vi "PythonIDE 2.vi"(7 "Python version":string="3.9", 11 "Port":string) -> ()   [LabVIEW 2020]
uses:
  <vilib>/event_ctls.llb/eventvkey.ctl
  <vilib>/Utility/error.llb/DialogType.ctl
  Serial_Global.vi
panel:
  out "VKey":T1
  out "message":string=" INSTRUCTIONS:\r\rNormal Use:  When using subVIs that incorporate the error in/error out (or error I/O) structure, place this handler where you want to inform the user of an error, typically at the end of the I/O data path, as the last action of the program.  If the error in error? is ERROR, the handler creates a message describing the error and its source.  If the type of dialog = 1 (default), the message is displayed to the user, who can only acknowedge it.  If the type = 2, the user can acknowledge the message or abort execution; aborting a program with active I/O is not recommended.  If the type = 0, no message is displayed; this is used to process the error programmatically, and the error out cluster elements are wired to individual terminals for that reason.  \r\rOther Use:\n\r\nlocal testing.  To test the error code of a subVI or function that does not have the error I/O structure, you can wire its error code and a source string to the local error code and error source inputs.  If error in error? indicates no error and error code is not equal to 0, the local code and source are substituted for the error in values, and error? is set TRUE (ERROR)."
  in  "Browser":bool
  in  "Name":string="code.py"
  in  "Save SPIKE":bool
  in  "Save PC":bool
  out "Script":string
  in  "Python Code":string
  out "Console":string
  in  "stop":bool
  in  "Ctrl C":bool
  in  "run":bool
  # "PyVIEW IDE\nversion 0.1b03"
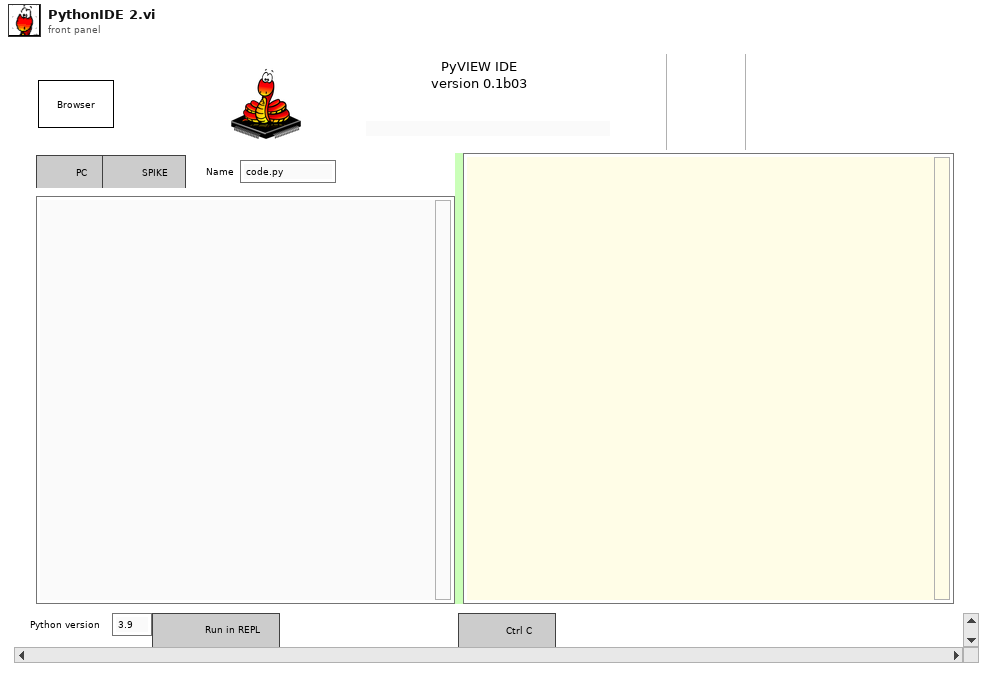
[diagram p1: front panel]
types:
  T1 = typedef "eventvkey.ctl" = enum16{"ASCII", "Enter", "Return", "Shift", "Ctrl", "Alt", "Cmd", "Opt", "Caps", "NumLock", "Clear", "Break", "Up", "Down", "Left", "Right", "Insert", "Delete", "Home", "End", "PageUp", "PageDown", "Escape", "Help", "Pause", "ScrollLock", "F1", "F2", "F3", "F4", "F5", "F6", "F7", "F8", "F9", "F10", "F11", "F12", "F13", "F14", "F15", "F16", "F17", "F18", "F19", "F20", "F21", "F22", "F23", "F24", "Play", "VolumeUp", "VolumeDown", "Mute", "Two Byte Char"}
  T2 = typedef "PythonCtrl.ctl" = cluster{"session":refnum<k35>, "PyPath":path}
  T3 = typedef "DialogType.ctl" = u16
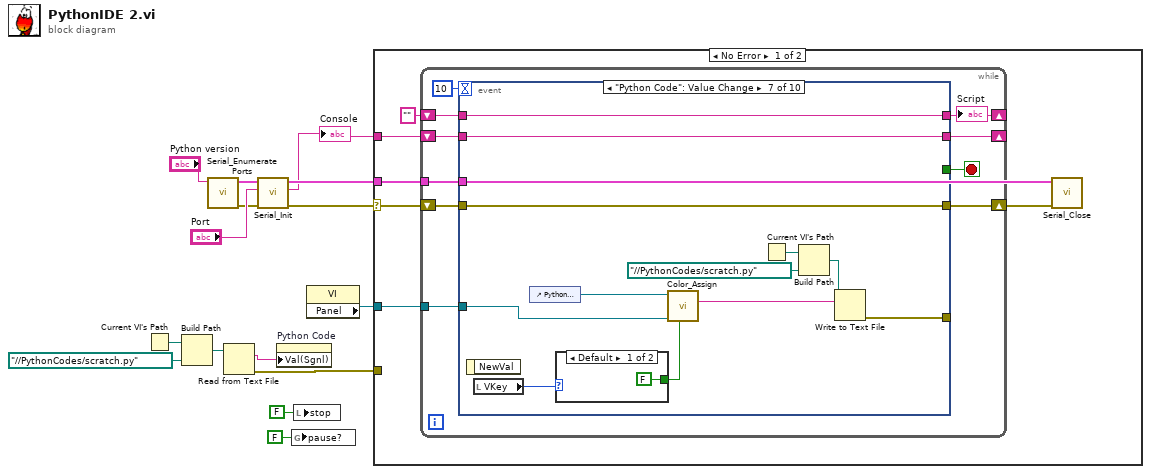
[diagram p0: block diagram]
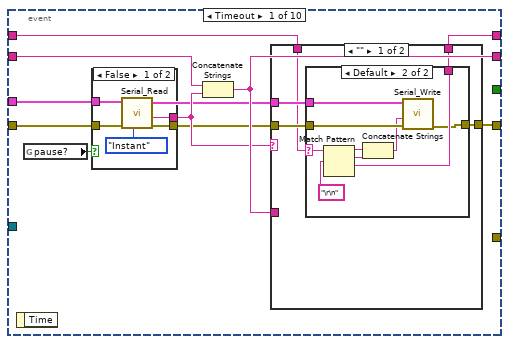
[diagram p2: hidden frame]
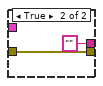
[diagram p3: hidden frame]
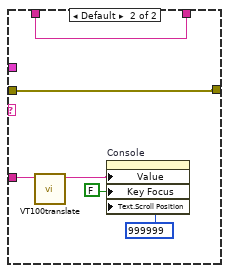
[diagram p5: hidden frame]
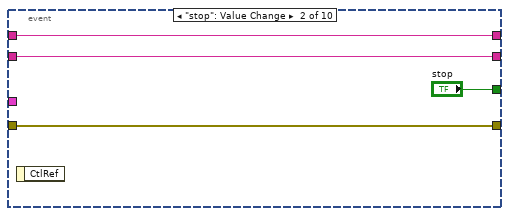
[diagram p6: hidden frame]
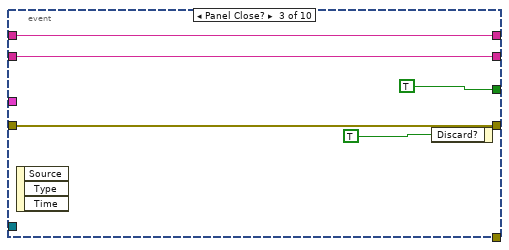
[diagram p7: hidden frame]
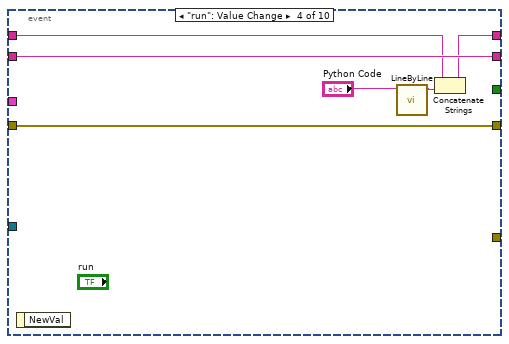
[diagram p8: hidden frame]
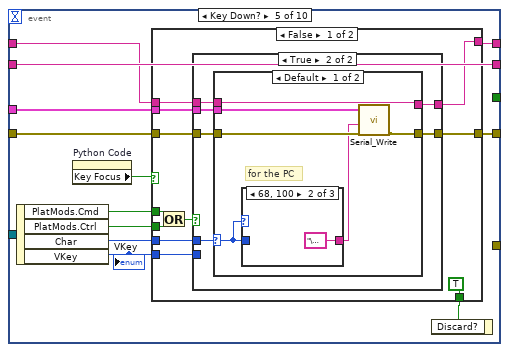
[diagram p9: hidden frame]
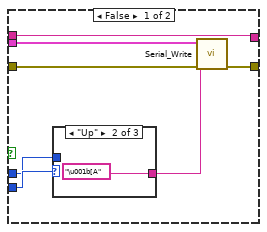
[diagram p10: hidden frame]
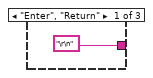
[diagram p11: hidden frame]
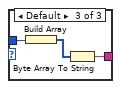
[diagram p12: hidden frame]
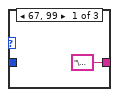
[diagram p13: hidden frame]
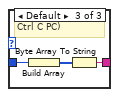
[diagram p14: hidden frame]
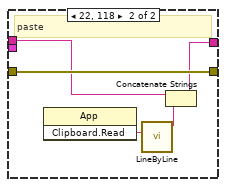
[diagram p15: hidden frame]
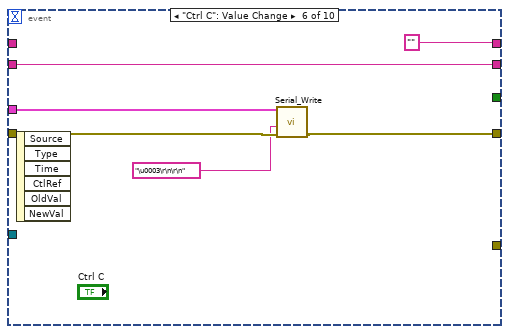
[diagram p18: hidden frame]
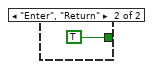
[diagram p19: hidden frame]
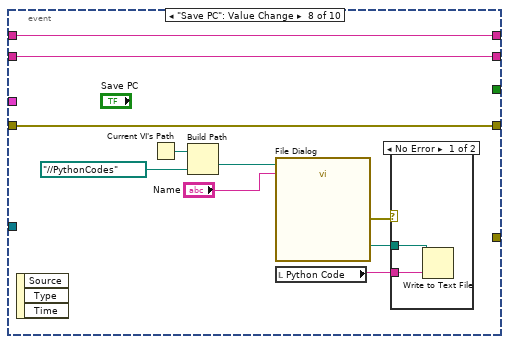
[diagram p20: hidden frame]
diagram:
  n1 = Current VI's Path() -> (path=w5:path)
  n2 = Build Path(base path=w5, name or relative path=path "../../PythonCodes/scratch.py") -> (appended path=w4:path)
  n3 = call "Serial_Enumerate Ports.vi"("Python version"="Python version") -> ("error out"=w9:errorcluster, "Python"=w11:T2)  [unwired: 7 in, 2 out]
  n4 = Read from Text File(file (use dialog)=w4) -> (text=w2:string, error out=w3:errorcluster)  [unwired: 3 in, 2 out]
  n5 = call "Serial_Init.vi"("error in (no error)"=w9, "Port"="Port", "Python"=w11) -> ("error out"=w7:errorcluster, "Console"=w8:string, "Python out"=w10:T2)  [unwired: 6 in]
  "Console" <- w8
  n6 = property on="Python Code" class="Str"("Val(Sgnl)"=w2) -> ()  [unwired: 2 in, 2 out]
  n7 = global write "Serial_Global.vi" "pause?"(FALSE ("pause?")) -> ()
  n8 = local write "stop"(FALSE ("stop")) -> ()
  n9 = property class="VI"() -> ("Panel"=w12:refnum<vi>)  [unwired: 2 in, 2 out]
  n10 = case shown="No Error" w7 {
    selector: w7 -> [w20 w199]
    tunnel: w12 -> [w21 _]
    tunnel: w8 -> [w18 _]
    tunnel: w10 -> [w17 _]
    tunnel: w3 -> [_ _]
    frame No Error {
      n11 = while {
        shift-right: [w30] -> _
        shift-left: w18 -> [w31]
        shift-right: [w26] -> w16
        shift-left: w20 -> [w27]
        tunnel: w21 -> [w25]
        shift-right: [w23] -> _
        shift-left: "" -> [w24]
        tunnel: w17 -> [w22]
        stop <- w29 stop-if-true
        n12 = event shown="[6] \"Python Code\": Value Change" {
          selector: _ -> [_ _ _ _ _ _ _ _ _ _]
          dyn-events: _ -> [_ _ _ _ _ _ _ _ _ _]
          timeout: 10 -> [_ _ _ _ _ _ _ _ _ _]
          tunnel: w22 -> [w33 _ _ _ w97 w150 _ _ w183 _]
          tunnel: w31 -> [w41 w73 w79 w85 w96 w151 w163 w174 w180 w196]
          tunnel: [w40 w73 w79 w85 w96 w151 w163 w174 w180 w196] -> w30
          tunnel: [_ "stop" TRUE ("stop") _ _ _ _ _ _ _] -> w29
          tunnel: w27 -> [w36 w72 w78 w84 w90 w149 w162 w173 w182 w197]
          tunnel: [w39 w72 w78 w84 w91 w147 w162 w173 w181 w197] -> w26
          tunnel: w25 -> [_ _ _ _ _ _ w161 _ _ _]
          tunnel: [w38 w71 w75 w82 w86 "" w160 w175 w184 w195] -> w23
          tunnel: w24 -> [w37 w71 w75 w83 w87 _ w160 w175 w184 w195]
          tunnel: [_ _ _ _ _ _ w156 _ _ _] -> _
          event Timeout {
            n13 = event-data() -> ()  [unwired: 1 in, 1 out]
            n14 = global read "Serial_Global.vi" "pause?"() -> (w32:bool)
            n15 = case shown="False" w32 {
              tunnel: w36 -> [w46 w48]
              tunnel: [w45 "" ("Text read")] -> w35
              tunnel: [w44 w48] -> w34
              tunnel: w33 -> [w43 _]
              frame False {
                n16 = call "Serial_Read.vi"("Task"=enum16{"Instant", "All"}."Instant", "error in (no error)"=w46, "Python"=w43) -> ("error out"=w44:errorcluster, "Text read"=w45:string)  [unwired: 7 in]
              }
              frame True {
              }
            }
            n17 = Concatenate Strings(w41, w35) -> (w40:string)
            n18 = case shown="\"\"" w35 {
              tunnel: w40 -> [_ w70]
              tunnel: w34 -> [w52 w66]
              tunnel: [w51 w66] -> w39
              tunnel: w37 -> [w49 w65]
              tunnel: [w53 w65] -> w38
              tunnel: w33 -> [w50 _]
              frame "" {
                n19 = case shown="Default" w49 {
                  selector: w49 -> [w55 w56]
                  tunnel: [w55 w64] -> w53
                  tunnel: w52 -> [w54 w60]
                  tunnel: [w54 w59] -> w51
                  tunnel: w50 -> [_ w57]
                  frame "" {
                  }
                  frame Default {
                    n20 = Match Pattern(string=w56, regular expression="\r\n") -> (before substring=w62:string, match substring=w61:string, after substring=w64:string)  [unwired: 1 in, 1 out]
                    n21 = Concatenate Strings(w62, w61) -> (w58:string)
                    n22 = call "Serial_Write.vi"("error in (no error)"=w60, "Text to write"=w58, "Python"=w57) -> ("error out"=w59:errorcluster)  [unwired: 8 in]
                  }
                }
              }
              frame Default {
                n23 = call "VT100translate.vi"("Console"=w70) -> ("Console 2"=w68:string)  [unwired: 10 in]
                n24 = property on="Console" class="Str"("Value"=w68, "Key Focus"=FALSE, "Text.Scroll Position"=u32 999999) -> ()  [unwired: 2 in, 2 out]
              }
            }
          }
          event "stop": Value Change {
            n25 = event-data() -> ()  [unwired: 1 in, 1 out]
          }
          event Panel Close? {
            n26 = event-data() -> ()  [unwired: 1 in, 3 out]
            n27 = event-data("Discard?"=TRUE ("stop")) -> ()  [unwired: 1 in, 1 out]
          }
          event "run": Value Change {
            n28 = event-data() -> ()  [unwired: 1 in, 1 out]
            n29 = call "LineByLine.vi"("Python Code"="Python Code") -> ("result string"=w81:string)  [unwired: 10 in]
            n30 = Concatenate Strings(w83, w81) -> (w82:string)
          }
          event Key Down? {
            n31 = event-data() -> ("PlatMods.Cmd"=w92:bool, "PlatMods.Ctrl"=w93:bool, "Char"=w94:i16, "VKey"=w95:T1)  [unwired: 1 in]
            "VKey" <- w95
            n32 = property on="Python Code" class="Str"() -> ("Key Focus"=w88:bool)  [unwired: 2 in, 2 out]
            n33 = case shown="False" w88 {
              tunnel: w97 -> [w102 _]
              tunnel: w95 -> [w108 _]
              tunnel: w94 -> [w107 w144]
              tunnel: w93 -> [w106 _]
              tunnel: w92 -> [w105 _]
              tunnel: [w100 w145] -> w91
              tunnel: w90 -> [w101 w145]
              tunnel: [TRUE ("Discard?") _] -> w89
              tunnel: w87 -> [w99 w143]
              tunnel: [w98 w143] -> w86
              frame False {
                n34 = Or(x=w105, y=w106) -> (x .or. y?=w104:bool)
                n35 = case shown="True" w104 {
                  tunnel: w108 -> [w115 _]
                  tunnel: w107 -> [w114 w126]
                  tunnel: w102 -> [w113 w125]
                  tunnel: w101 -> [w112 w124]
                  tunnel: [w110 w123] -> w100
                  tunnel: w99 -> [w109 w122]
                  tunnel: [w109 w121] -> w98
                  frame False {
                    n36 = case shown="\"Up\"" w115 {
                      tunnel: w114 -> [_ _ w120]
                      tunnel: ["\r\n" ("replace string (\"\")") "\u001b[A" ("replace string (\"\")") w118] -> w111
                      frame "Enter", "Return" {
                      }
                      frame "Up" {
                      }
                      frame Default {
                        n37 = Build Array(w120) -> (w119:i16[])
                        n38 = Byte Array To String(unsigned byte array=w119) -> (string=w118:string)
                      }
                    }
                    n39 = call "Serial_Write.vi"("error in (no error)"=w112, "Text to write"=w111, "Python"=w113) -> ("error out"=w110:errorcluster)  [unwired: 8 in]
                  }
                  frame True {
                    n40 = case shown="Default" w126 {
                      selector: w126 -> [w127 _]
                      tunnel: w125 -> [w132 _]
                      tunnel: w124 -> [w131 w142]
                      tunnel: [w130 w142] -> w123
                      tunnel: w122 -> [w128 w141]
                      tunnel: [w128 w140] -> w121
                      frame Default {
                        # "for the PC"
                        n41 = case shown="68, 100" w127 {
                          tunnel: w127 -> [_ _ w136]
                          tunnel: ["\u0003" ("string") "\u0004" ("string") w135] -> w129
                          frame 67, 99 {
                          }
                          frame 68, 100 {
                          }
                          frame Default {
                            # "Ctrl C PC)"
                            n42 = Build Array(w136) -> (w137:i16[])
                            n43 = Byte Array To String(unsigned byte array=w137) -> (string=w135:string)
                          }
                        }
                        n44 = call "Serial_Write.vi"("error in (no error)"=w131, "Text to write"=w129, "Python"=w132) -> ("error out"=w130:errorcluster)  [unwired: 8 in]
                      }
                      frame 22, 118 {
                        # "paste"
                        n45 = invoke class="App" method="Clipboard.Read"() -> ("Read Clipbrd"=w139:string)  [unwired: 3 in, 2 out]
                        n46 = call "LineByLine.vi"("Python Code"=w139) -> ("result string"=w138:string)  [unwired: 10 in]
                        n47 = Concatenate Strings(w141, w138) -> (w140:string)
                      }
                    }
                  }
                }
              }
              frame True {
                n48 = case shown="1" w144 {
                  frame 0, Default {
                  }
                  frame 1 {
                  }
                }
              }
            }
            n49 = event-data("Discard?"=w89) -> ()  [unwired: 1 in, 1 out]
          }
          event "Ctrl C": Value Change {
            n50 = event-data() -> ()  [unwired: 1 in, 6 out]
            n51 = call "Serial_Write.vi"("error in (no error)"=w149, "Text to write"="\u0003\r\n\r\n" ("function name"), "Python"=w150) -> ("error out"=w147:errorcluster)  [unwired: 8 in]
          }
          event "Python Code": Value Change {
            n52 = event-data() -> ()  [unwired: 1 in, 1 out]
            n53 = local read "VKey"() -> (w154:T1)
            n54 = control-ref of="Python Code"() -> (w155:refnum<vi>)
            n55 = case shown="Default" w154 {
              tunnel: [FALSE TRUE] -> w153
              frame Default {
              }
              frame "Enter", "Return" {
              }
            }
            n56 = call "Color_Assign.vi"("Add Spaces?"=w153, "Front Panel"=w161, "Code"=w155) -> ("Value"=w152:string)  [unwired: 8 in]
            n57 = Current VI's Path() -> (path=w159:path)
            n58 = Build Path(base path=w159, name or relative path=path "../../PythonCodes/scratch.py") -> (appended path=w157:path)
            n59 = Write to Text File(file (use dialog)=w157, text=w152) -> (error out=w156:errorcluster)  [unwired: 2 in, 2 out]
          }
          event "Save PC": Value Change {
            n60 = event-data() -> ()  [unwired: 1 in, 3 out]
            n61 = Current VI's Path() -> (path=w171:path)
            n62 = Build Path(base path=w171, name or relative path=path "../../PythonCodes") -> (appended path=w168:path)
            n63 = call "File Dialog"("start path"=w168, "default name"="Name") -> ("selected path"=w167:path, "error out"=w166:errorcluster)  [unwired: 10 in, 2 out]
            n64 = local read "Python Code"() -> (w172:string)
            n65 = case shown="No Error" w166 {
              tunnel: w172 -> [w177 _]
              tunnel: w167 -> [w176 _]
              frame No Error {
                n66 = Write to Text File(file (use dialog)=w176, text=w177) -> ()  [unwired: 2 in, 3 out]
              }
              frame Error {
              }
            }
          }
          event "Save SPIKE": Value Change {
            n67 = event-data() -> ()  [unwired: 1 in, 3 out]
            n68 = local read "Python Code"() -> (w178:string)
            n69 = local read "Name"() -> (w179:string)
            n70 = call "ReadFileDialog.vi"("File Text"=w178, "error in (no error)"=w182, "File name"=w179, "Python in"=w183) -> ("error out"=w181:errorcluster)  [unwired: 6 in, 1 out]
          }
          event "Browser": Value Change {
            w193 = 128  # call and forget
            n71 = event-data() -> ()  [unwired: 1 in, 3 out]
            n72 = vi-ref "Examples.vi"() -> (w190:refnum<vi>)
            n73 = property class="VI"(reference=w190) -> ("Name"=w191:string)  [unwired: 1 in, 2 out]
            n74 = local read "Port"() -> (w189:string)
            n75 = Open VI Reference(type specifier VI Refnum (for type only)=refnum<vi> refnum, vi path=w191, options=w193) -> (vi reference=w194:refnum<vi>, error out=w185:errorcluster)  [unwired: 3 in]
            n76 = local read "Python version"() -> (w188:string)
            n77 = call-by-ref "Start Asynchronous Call"(reference=w194, error in=w185, "Python version"=w188, "Port"=w189) -> (reference out=w186:refnum<vi>, error out=w187:errorcluster)  [unwired: 10 in]
            n78 = Close Reference(reference=w186, error in (no error)=w187) -> ()  [unwired: 1 out]
          }
        }
        "Script" <- w23
      }
      n79 = call "Serial_Close.vi"("error in (no error)"=w16, "Python in"=w17) -> ()  [unwired: 10 in]
    }
    frame Error {
      n80 = Unbundle By Name(w199) -> ("code"=w198:i32)
      n81 = case shown="1671" w198 {
        tunnel: w199 -> [w209 w214]
        frame 1671 {
          w208 = T3 0 items=["no dialog", "OK message", "continue or stop message", "OK message + warnings", "continue/stop + warnings"] ("type of dialog (OK msg:1)")
          n82 = call <vilib>:"Simple Error Handler.vi"("type of dialog (OK msg:1)"=w208, "error in (no error)"=w209) -> ("message"=w207:string)  [unwired: 3 in, 4 out]
          n83 = Match Pattern(string=w207, regular expression="Function Name:") -> (after substring=w201:string)  [unwired: 1 in, 3 out]
          n84 = Match Pattern(string=w201, regular expression="\n\n") -> (before substring=w200:string)  [unwired: 1 in, 3 out]
          "message" <- w200
          n85 = Match Pattern(string=w201, regular expression="\n") -> (before substring=w204:string)  [unwired: 1 in, 3 out]
          n86 = call <vilib>:"Trim Whitespace.vi"("string"=w204) -> ("trimmed string"=w203:string)  [unwired: 1 in]
          n87 = case shown="\"InitSerial\"" w203 {
            tunnel: w200 -> [w211 _]
            frame Default {
              n88 = Concatenate Strings("Error in ", w211) -> (w210:string)
              n89 = One Button Dialog(message=w210) -> ()  [unwired: 1 in, 1 out]
            }
            frame "InitSerial" {
              n90 = One Button Dialog(message="Could not initialize serial port - try selecting a different one.") -> ()  [unwired: 1 in, 1 out]
            }
          }
        }
        frame Default {
          n91 = call <vilib>:"Simple Error Handler.vi"("error in (no error)"=w214) -> ()  [unwired: 4 in, 5 out]
        }
      }
    }
  }
